vi "zSpec_trigger.vi"(7 "Error in (no error)":errorcluster, 8 "trigger 2":sgl format="%#_6p", 9 "trigger1":sgl=-5.0 format="%#_6p", 10 "Application ref in":refnum<vi>) -> (0 "Error out":errorcluster, 3 "Application ref out":refnum<vi>)   [LabVIEW 2021]
uses:
  <userlib>/Nanonis Prog Interface V5/Nanonis Prog Interface.lvlib
panel:
  out "trigger2":bool
  out "trigger1":bool=TRUE
  in  "integration":i32=6
  in  "Oversampling (10)":i32=1
  out "Signal value":sgl=-4.159982 format="%#_6p"
  in  "Animations Period (s)":sgl=0.005 format="%#_6p"
  in  "Ring":u16(ring)=50 items=["Current (A)", "Input 2 (V)", "T-Cryo (K)", "T-STM (K)", "Input 5 (V)", "Input 6 (V)", "Input 7 (V)", "Input 8 (V)", "Input 9  (V)", "Input10  (V)", "Input11  (V)", "Input12  (V)", "Input13  (V)", "Input14  (V)", "Input15  (V)", "Input16  (V)", "Input17  (V)", "Input18  (V)", "Input19  (V)", "Input20  (V)", "Input21  (V)", "Input22  (V)", "Input23  (V)", "Input24  (V)", "Bias (V)", "Output 2 (A)", "TCryo Supply voltage (V)", "STM Supply voltage (V)", "X (m)", "Y (m)", "Z (m)", "Output 8 (V)", "Output 9  (V)", "Output10  (V)", "Output11  (V)", "Output12  (V)", "Output13  (V)", "Output14  (V)", "Output15  (V)", "Output16  (V)", "Output17  (V)", "Output18  (V)", "Output19  (V)", "Output20  (V)", "Output21  (V)", "Output22  (V)", "Output23  (V)", "Output24  (V)", "OC D1 Phase (deg)", "OC D1 Amplitude (m)", "OC M1 Freq. Shift (Hz)", "OC M1 Excitation (V)", "OC D1 X (m)", "OC D1 Y (m)", "OC D2 Phase (deg)", "OC D2 Amplitude (m)", "Reserved  9  (V)", "Reserved 10  (V)", "OC D2 X (m)", "OC D2 Y (m)", "LI Demod 1 X (A)", "LI Demod 1 Y (A)", "LI Demod 2 X (A)", "LI Demod 2 Y (A)", "Reserved 17  (V)", "Reserved 18  (V)", "Reserved 19  (V)", "Reserved 20  (V)", "Reserved 21  (V)", "Reserved 22  (V)", "Internal 23 (V)", "Internal 24 (V)", "Z Control signal (A)", "Z Error signal (A)", "Z SafeTip signal (A)", "Reserved 28  (V)", "OC D3 Amplitude (m)", "OC D3 Phase (deg)", "OC D4 Amplitude (m)", "OC D4 Phase (deg)"]
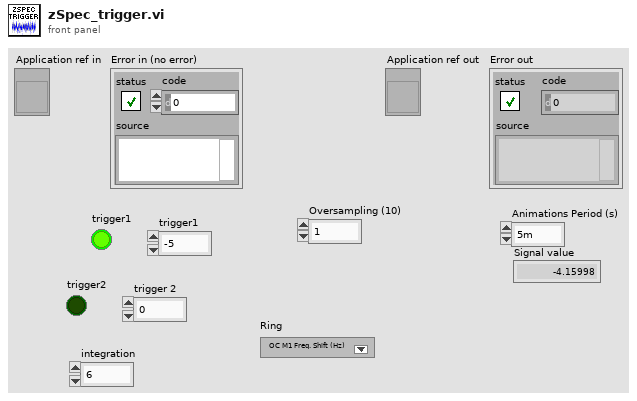
[diagram p1: front panel]
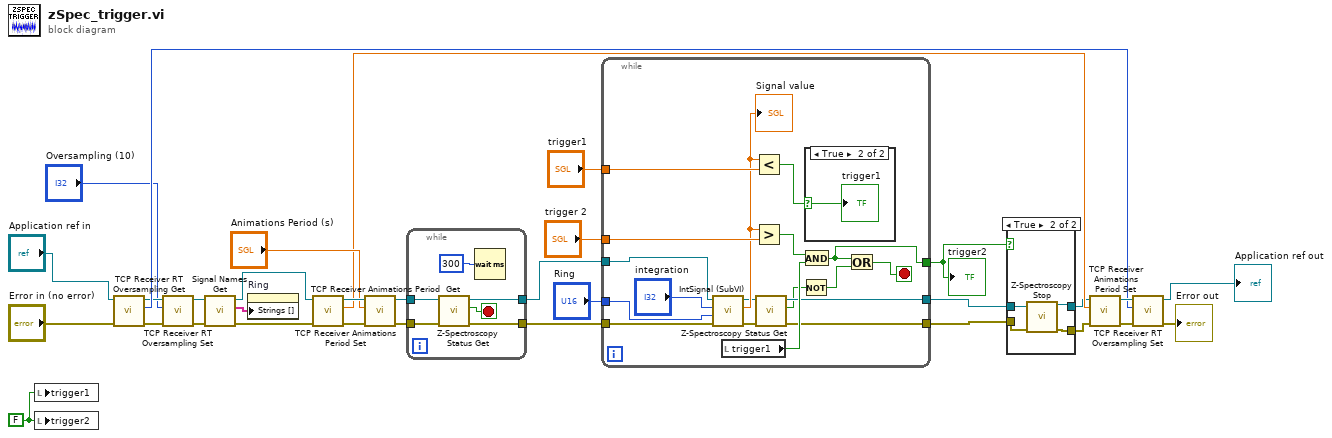
[diagram p0: block diagram]
diagram:
  w10 = FALSE ("trigger1")
  n1 = local write "trigger1"(w10) -> ()
  n2 = local write "trigger2"(w10) -> ()
  n3 = call <userlib>:"TCP Receiver RT Oversampling Get.vi"("Error in (no error)"="Error in (no error)", "Application ref in"="Application ref in") -> ("Error out"=w19:errorcluster, "Oversampling"=w23:i32, "Application ref out"=w21:refnum<vi>)  [unwired: 7 in]
  n4 = call <userlib>:"TCP Receiver RT Oversampling Set.vi"("Error in (no error)"=w19, "Oversampling (10)"="Oversampling (10)", "Application ref in"=w21) -> ("Error out"=w18:errorcluster, "Application ref out"=w20:refnum<vi>)  [unwired: 7 in]
  n5 = call <userlib>:"Signal Names Get.vi"("error in (no error)"=w18, "Application ref in"=w20) -> ("error out"=w31:errorcluster, "Signals Names"=w32:string[], "Application ref out"=w30:refnum<vi>)  [unwired: 5 in]
  n6 = property on="Ring" class="Ring (strict)"("Strings []"=w32) -> ()  [unwired: 2 in, 2 out]
  n7 = call <userlib>:"TCP Receiver Animations Period  Get.vi"("Error in (no error)"=w31, "Application ref in"=w30) -> ("Error out"=w29:errorcluster, "Animations Period (s)"=w22:sgl, "Application ref out"=w28:refnum<vi>)  [unwired: 7 in]
  n8 = call <userlib>:"TCP Receiver Animations Period Set.vi"("Error in (no error)"=w29, "Animations Period (s)"="Animations Period (s)", "Application ref in"=w28) -> ("Error out"=w3:errorcluster, "Application ref out"=w5:refnum<vi>)  [unwired: 7 in]
  n9 = while {
    tunnel: w5 -> [w38]
    tunnel: [w37] -> w4
    tunnel: w3 -> [w36]
    tunnel: [w35] -> w2
    stop <- w34 stop-if-true
    n10 = call <userlib>:"Z-Spectroscopy Status Get.vi"("Error in (no error)"=w36, "Application ref in"=w38) -> ("Error out"=w35:errorcluster, "Running?"=w34:bool, "Application ref out"=w37:refnum<vi>)  [unwired: 5 in]
    n11 = Wait (ms)(milliseconds to wait=u32 300) -> ()  [unwired: 1 out]
  }
  n12 = while {
    tunnel: "Ring" -> [w56]
    tunnel: w4 -> [w55]
    tunnel: w2 -> [w54]
    tunnel: [w45] -> w15
    tunnel: [w43] -> w12
    tunnel: "trigger1" -> [w53]
    tunnel: "trigger 2" -> [w50]
    tunnel: [w39] -> w6
    stop <- w41 stop-if-true
    n13 = call "IntSignal (SubVI).vi"("error in (no error)"=w54, "channel"=w56, "integration"="integration", "Application in"=w55) -> ("error out"=w44:errorcluster, "Signal value"=w49:sgl, "Application out"=w46:refnum<vi>)  [unwired: 5 in]
    "Signal value" <- w49
    n14 = local read "trigger1"() -> (w47:bool)
    n15 = Less?(x=w49, y=w53) -> (x < y?=w51:bool)
    n16 = Greater?(x=w49, y=w50) -> (0:w48:bool)
    n17 = call <userlib>:"Z-Spectroscopy Status Get.vi"("Error in (no error)"=w44, "Application ref in"=w46) -> ("Error out"=w43:errorcluster, "Running?"=w42:bool, "Application ref out"=w45:refnum<vi>)  [unwired: 5 in]
    n18 = Not(x=w42) -> (.not. x?=w40:bool)
    n19 = And(x=w48, y=w47) -> (x .and. y?=w39:bool)
    n20 = case shown="True" w51 {
      selector: w51 -> [_ w57]
      frame False {
      }
      frame True {
        "trigger1" <- w57
      }
    }
    n21 = Or(x=w39, y=w40) -> (x .or. y?=w41:bool)
  }
  "trigger2" <- w6
  n22 = case shown="True" w6 {
    tunnel: w15 -> [w58 w63]
    tunnel: [w58 w60] -> w14
    tunnel: [w59 w61] -> w13
    tunnel: w12 -> [w59 w62]
    frame False {
    }
    frame True {
      n23 = call <userlib>:"Z-Spectroscopy Stop.vi"("Application ref in"=w63, "Error in (no error)"=w62) -> ("Application ref out"=w60:refnum<vi>, "Error out"=w61:errorcluster)  [unwired: 12 in]
    }
  }
  n24 = call <userlib>:"TCP Receiver Animations Period Set.vi"("Error in (no error)"=w13, "Animations Period (s)"=w22, "Application ref in"=w14) -> ("Error out"=w25:errorcluster, "Application ref out"=w24:refnum<vi>)  [unwired: 7 in]
  n25 = call <userlib>:"TCP Receiver RT Oversampling Set.vi"("Error in (no error)"=w25, "Oversampling (10)"=w23, "Application ref in"=w24) -> ("Error out"=→"Error out":errorcluster, "Application ref out"=→"Application ref out":refnum<vi>)  [unwired: 7 in]
